vi "File_SaveVIUniqueName.vi"(8 "error in (no error)":errorcluster, 9 "Save a Copy":bool, 10 "appended path":path, 11 "VI in":refnum<vi>) -> (0 "error out":errorcluster, 2 "NewName":path, 3 "VI out":refnum<vi>)   [LabVIEW 2014]
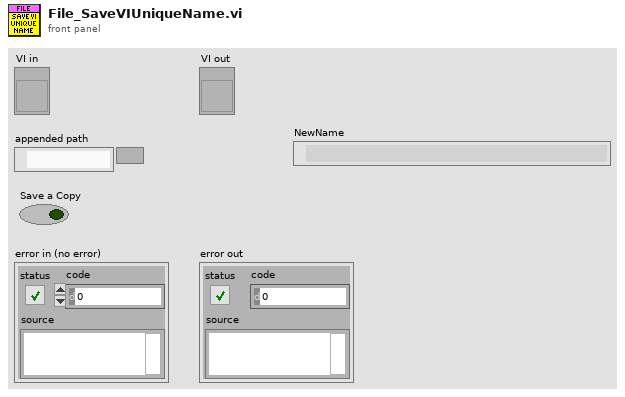
[diagram p1: front panel]
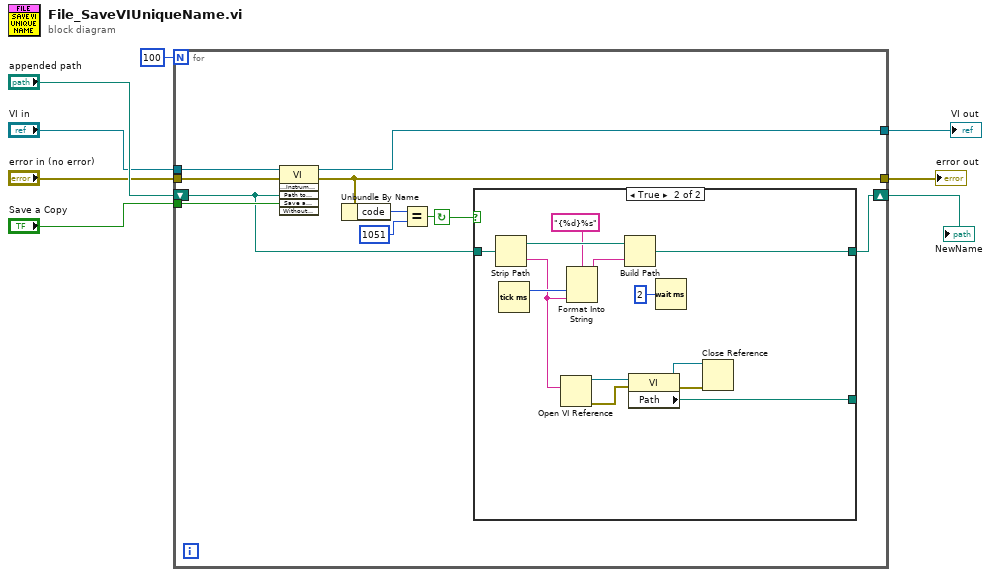
[diagram p0: block diagram]
diagram:
  n1 = for {
    N: 100 -> [_]
    tunnel: [w14] -> w7
    tunnel: [w18] -> w6
    tunnel: "Save a Copy" -> [w17]
    tunnel: "error in (no error)" -> [w16]
    tunnel: "VI in" -> [w15]
    shift-right: [w9] -> w1
    shift-left: "appended path" -> [w10]
    stop <- w11 continue-if-true
    n2 = invoke class="VI" method="Save.Instrument"(reference=w15, error in=w16, "Path to saved file"=w10, "Save a Copy"=w17) -> (reference out=w18:refnum<vi>, error out=w14:errorcluster)  [unwired: 2 in, 4 out]
    n3 = Unbundle By Name(w14) -> ("code"=w13:i32)
    n4 = Equal?(x=w13, y=1051) -> (x = y?=w11:bool)
    n5 = case shown="True" w11 {
      tunnel: w10 -> [w19 w32]
      tunnel: [w19 w27] -> w9
      tunnel: [_ w22] -> _
      frame False {
      }
      frame True {
        n6 = Strip Path(path=w32) -> (stripped path=w31:path, name=w25:string)
        n7 = Tick Count (ms)() -> (millisecond timer value=w30:u32)
        n8 = Open VI Reference(vi path=w25) -> (vi reference=w24:refnum<vi>, error out=w23:errorcluster)  [unwired: 5 in]
        n9 = Format Into String(format string="{%d}%s" ("resulting string"), w30, w25) -> (resulting string=w29:string)  [unwired: 2 in, 1 out]
        n10 = Build Path(base path=w31, name or relative path=w29) -> (appended path=w27:path)
        n11 = property class="VI"(reference=w24, error in=w23) -> (reference out=w20:refnum<vi>, error out=w21:errorcluster, "Path"=w22:path)
        n12 = Wait (ms)(milliseconds to wait=u32 2) -> ()  [unwired: 1 out]
        n13 = Close Reference(reference=w20, error in (no error)=w21) -> ()  [unwired: 1 out]
      }
    }
  }
  "error out" <- w7
  "VI out" <- w6
  "NewName" <- w1
